vi "AssertSubpanelVIExecBad.vi"(0 "VI Reference In":refnum<vi>, 1 "Test Label":string, 2 "delimiter (>>)":string=">>", 3 "Assert Only? (F)":bool, 5 "Control Path":string, 11 "Error In":errorcluster, 12 "Assert Interval(10 ms)":u32=10, 13 "Timeout(5 sec)":dbl=5.0) -> (4 "VI Reference Out":refnum<vi>, 6 "Asserted Value":T1(ring), 15 "Error Out":errorcluster)   [LabVIEW 2016, in "Drona.lvlib" / "AssertControlValue.lvlib" / "AssertSubpanel.lvlib"]
doc: "Asserts if the Inserted VI in Subpanel is in Bad execution state.\nThe input control name is given as a string , incase of path, use delimiters inbetween the path."
uses:
  AssertSubpanel.lvlib
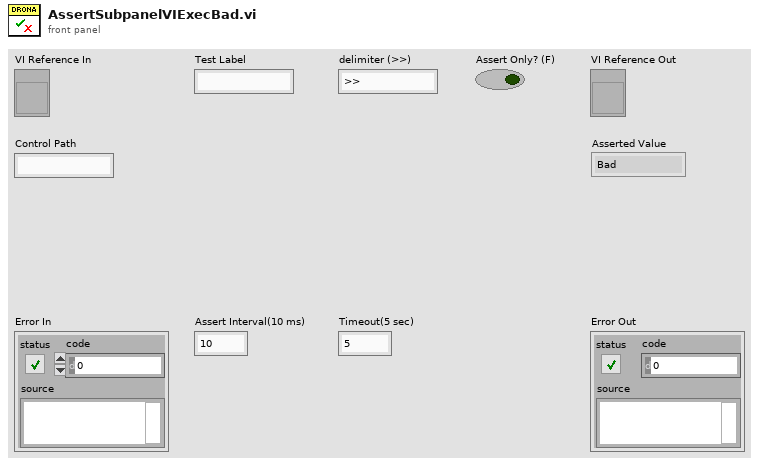
[diagram p1: front panel]
types:
  T1 = enum32{"Bad", "Idle", "Run top level", "Running"}
  T2 = enum32{"Bad", "Idle", "Run top level", "Running"}[]
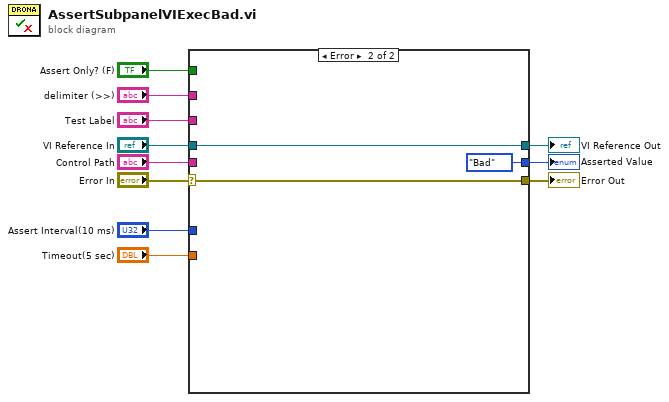
[diagram p0: block diagram]
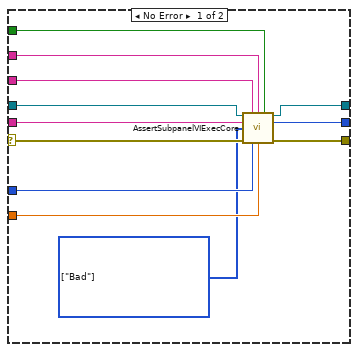
[diagram p2: hidden frame]
diagram:
  n1 = case shown="Error" "Error In" {
    selector: "Error In" -> [w22 w26]
    tunnel: [w23 w26] -> w11
    tunnel: "Timeout(5 sec)" -> [w21 _]
    tunnel: [w20 w25] -> w8
    tunnel: "Assert Interval(10 ms)" -> [w19 _]
    tunnel: "Test Label" -> [w18 _]
    tunnel: "Control Path" -> [w17 _]
    tunnel: "delimiter (>>)" -> [w16 _]
    tunnel: "Assert Only? (F)" -> [w15 _]
    tunnel: "VI Reference In" -> [w13 w25]
    tunnel: [w12 T1."Bad" ("Asserted Value")] -> w1
    frame No Error {
      w14 = T2 [enum."Bad"] items=["Bad", "Idle", "Run top level", "Running"] ("Execution:State")
      n2 = call "AssertSubpanelVIExecCore.vi"("VI Reference In"=w13, "Label"=w18, "delimiter (>>)"=w16, "Assert Only? (F)"=w15, "Control Path"=w17, "Execution:State"=w14, "Error In"=w22, "Assert Interval(10 ms)"=w19, "Timeout(5 sec)"=w21) -> ("VI Reference Out"=w20:refnum<vi>, "Asserted Value"=w12:T1, "Error Out"=w23:errorcluster)  [unwired: 4 in]
    }
    frame Error {
    }
  }
  "Error Out" <- w11
  "VI Reference Out" <- w8
  "Asserted Value" <- w1
